vi "未命名 4.vi"() -> ()   [LabVIEW 2017]
panel:
  out "y":dbl
  in  "b":dbl
  in  "x":dbl
  in  "k":dbl
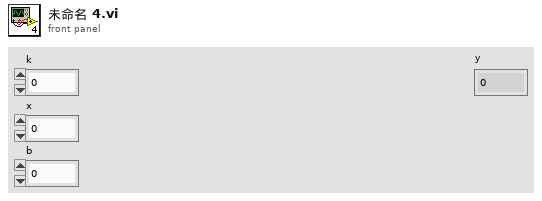
[diagram p1: front panel]
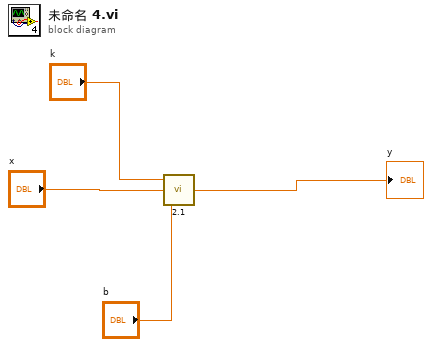
[diagram p0: block diagram]
diagram:
  n1 = call "2.1.vi"("b"="b", "x"="x", "k"="k") -> ("y"=→"y":dbl)
